vi "Read Tx Value.vi"(8 "error in (no error)":errorcluster, 11 "RxTx in":refnum<class "RxTx.lvclass">) -> (0 "error out":errorcluster, 2 "Tx Value":string, 3 "RxTx out":refnum<class "RxTx.lvclass">)   [LabVIEW 2018, in "RxTx.lvclass"]
uses:
  RxTx.lvclass
  RxTx.lvclass/RxTx.ctl
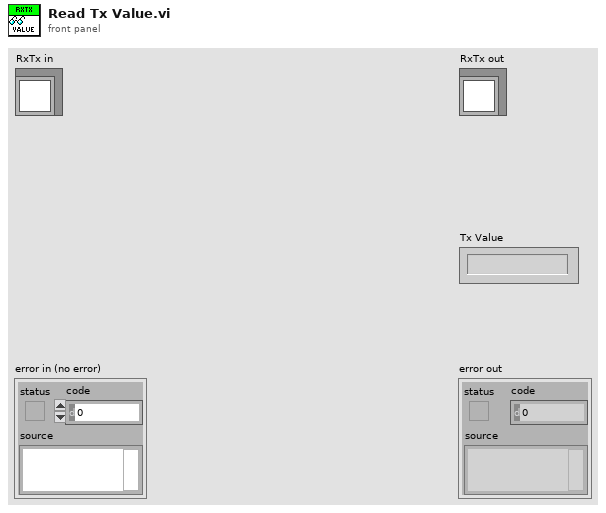
[diagram p1: front panel]
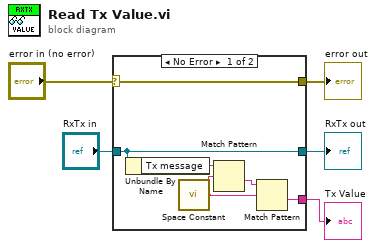
[diagram p0: block diagram]
diagram:
  n1 = case shown="No Error" "error in (no error)" {
    selector: "error in (no error)" -> [w11 w13]
    tunnel: [w11 w13] -> w4
    tunnel: [w10 w12] -> w2
    tunnel: "RxTx in" -> [w10 w12]
    tunnel: [w7 _] -> w1
    frame No Error {
      n2 = Unbundle By Name(w10) -> ("Tx message"=w9:string)
      n3 = call <vilib>:"Space Constant.vi"() -> ("String"=w6:string)
      n4 = Match Pattern(string=w9, regular expression=w6) -> (after substring=w8:string)  [unwired: 1 in, 3 out]
      n5 = Match Pattern(string=w8, regular expression=w6) -> (after substring=w7:string)  [unwired: 1 in, 3 out]
    }
    frame Error {
    }
  }
  "error out" <- w4
  "RxTx out" <- w2
  "Tx Value" <- w1
